vi "CSMsettings_ut_test.vi"(8 "Error In":errorcluster, 11 "CSMinfo in":T3={"Общие сведения"={"Регистрационный номер заказа"="", "Идентификация (шифр) образца"="", "IMEI образца"="", "НД, устанавливающий требования"="", "Методы испытаний (измерений)"="", "Дата начала испытаний"="", "Дата завершения испытаний"=""}, "Климатические условия внешней среды"={"Температура окружающего воздуха"="", "Относительная влажность воздуха"="", "Атмосферное давление"=""}, "Окно с настройками"={"Режим звонка связь"=0, "Напряжение источника"=0, "Условия окружающей среды"=0, "Номер образца"=0, "Источник питания"=0, "Номер испытания"=0, "Режим звонка тональный модем"=0, "Количество итераций TM"=100.0, "Аутентификация"=0, "Колличество повторов измерений"=1.0, "Сим карта"=0, "VISA adress of CMW500"="", "Input attenuation"=1.0, "Output attenuation"=1.0, "Call Release Type"=0, "GSM Band"=0, "BCCH Channel Number"=0.0, "TCH Channel Number"=0.0, "Codec"=0, "AWGN"=0, "snrRatioInDb"=0.0, "GSM Fading"=0, "UL C/I ratio"=0, "Use a custom network ID"=FALSE, "MCC (Mobile Country Code)"=0.0, "MNC (Mobile Network Code)"=0.0, "NCC (Network Color Code)"=0.0, "MNC digit count"=0, "BCC (Base station Color Code)"=0.0, "LAC (Location Area Code)"=0.0, "RAC (Routing Area Code)"=0.0, "Cell Identity"=0.0, "Override UE ID"=FALSE, "MCC (UE Mobile Country Code)"=0.0, "MNC (UE Mobile Network Code)"=0.0, "MSIN (Mobile Subscription ID)"=0.0, "InputScaleFactor"=0, "OutputScaleFactor"=0, "Post MSD wave file playback 3GPP  26.269 \nEU_DTMF_tones"=FALSE, "Scenario"=0, "AlAckBehavior"=0, "PSAP listens for PUSH"=FALSE, "BCCH Channel Power"=0.0, "TCH Channel Power"=0.0}} {"Окно с настройками"."AlAckBehavior" items=["POSITIVE", "CLEAR_DOWN", "LOOP_BACK_MSD_PART"]; "Окно с настройками"."Scenario" items=["NORMAL", "NORMAL_IMMEDIATE_START", "TIMEOUT_T3", "ALLRV_REQ", "SUPPRESS_MSD", "SUPPRESS_ALACK", "SUPPRESS_SEND_MSD"]; "Окно с настройками"."OutputScaleFactor" items=["ONE", "QUARTER", "HALF", "TWO", "FOUR"]; "Окно с настройками"."InputScaleFactor" items=["ONE", "QUARTER", "HALF", "TWO", "FOUR"]; "Окно с настройками"."MNC digit count" items=["TWO", "THREE"]; "Окно с настройками"."UL C/I ratio" items=["Ci1Db", "Ci4Db", "Ci7Db", "Ci10Db", "Ci13Db", "Ci16Db"]; "Окно с настройками"."GSM Fading" items=["GsmFadingOff", "GsmEtsiTs103412DlFading", "GsmEtsiTs103412UlFading", "GsmEtsiTs103412DlUlFading"]; "Окно с настройками"."AWGN" items=["Off", "50MhzAwgn"]; "Окно с настройками"."Codec" items=["FRV2", "AMRH_GMSK_7K95", "AMRH_GMSK_7K40", "AMRH_GMSK_6K70", "AMRH_GMSK_5K90", "AMRH_GMSK_5K15", "AMRH_GMSK_4K75", "AMRF_GMSK_12K20", "AMRF_GMSK_10K20", "AMRF_GMSK_7K95", "AMRF_GMSK_7K40 ", "AMRF_GMSK_6K70", "AMRF_GMSK_5K90", "AMRF_GMSK_5K15", "AMRF_GMSK_4K75", "FRV1", "HRV1", "WAMR_GMSK_6K60", "WAMR_GMSK_8K85", "WAMR_GMSK_12K65"]; "Окно с настройками"."GSM Band" items=["GSM450", "GSM850", "GSM900", "GSM1800", "GSM1900"]; "Окно с настройками"."Call Release Type" items=["NormalRelease", "CallInterruption"]; "Окно с настройками"."Сим карта" items=["SIM", "eSIM"]; "Окно с настройками"."Колличество повторов измерений" min=1.0 max=100.0 format="%#_3g"; "Окно с настройками"."Аутентификация" items=["On", "Off"]; "Окно с настройками"."Режим звонка тональный модем" items=["Автоматически (AT) GEMALTO", "Автоматически (AT) SIMCOM", "Автоматически (AT) TELIT", "Автоматически (AT) PROGRESS", "Автоматически (AT) PROGRESS GREEN", "Автоматически (AT) PROGRESS BLUE", "Автоматически (реле)", "Вручную"]; "Окно с настройками"."Номер испытания" items=["1", "2", "3"]; "Окно с настройками"."Источник питания" items=["Не используется", "IT6332A"]; "Окно с настройками"."Номер образца" items=["1", "2", "3"]; "Окно с настройками"."Условия окружающей среды" items=["UnormTnorm", "UminTmin", "UmaxTmin", "UminTmax", "UmaxTmax", "TypeA", "TypeB"]; "Окно с настройками"."Напряжение источника" items=["12", "24"]; "Окно с настройками"."Режим звонка связь" items=["Автоматически (AT) GEMALTO", "Автоматически (AT) SIMCOM", "Автоматически (AT) TELIT", "Автоматически (AT) PROGRESS", "Автоматически (AT) PROGRESS GREEN", "Автоматически (AT) PROGRESS BLUE", "Автоматически (реле)", "Вручную"]}) -> (0 "Error Out":errorcluster, 3 "CSMinfo out":T3={"Общие сведения"={"Регистрационный номер заказа"="", "Идентификация (шифр) образца"="", "IMEI образца"="", "НД, устанавливающий требования"="", "Методы испытаний (измерений)"="", "Дата начала испытаний"="", "Дата завершения испытаний"=""}, "Климатические условия внешней среды"={"Температура окружающего воздуха"="", "Относительная влажность воздуха"="", "Атмосферное давление"=""}, "Окно с настройками"={"Режим звонка связь"=0, "Напряжение источника"=0, "Условия окружающей среды"=0, "Номер образца"=0, "Источник питания"=0, "Номер испытания"=0, "Режим звонка тональный модем"=0, "Количество итераций TM"=0.0, "Аутентификация"=0, "Колличество повторов измерений"=1.0, "Сим карта"=0, "VISA adress of CMW500"="", "Input attenuation"=1.0, "Output attenuation"=1.0, "Call Release Type"=0, "GSM Band"=0, "BCCH Channel Number"=0.0, "TCH Channel Number"=0.0, "Codec"=0, "AWGN"=0, "snrRatioInDb"=0.0, "GSM Fading"=0, "UL C/I ratio"=0, "Use a custom network ID"=FALSE, "MCC (Mobile Country Code)"=0.0, "MNC (Mobile Network Code)"=0.0, "NCC (Network Color Code)"=0.0, "MNC digit count"=0, "BCC (Base station Color Code)"=0.0, "LAC (Location Area Code)"=0.0, "RAC (Routing Area Code)"=0.0, "Cell Identity"=0.0, "Override UE ID"=FALSE, "MCC (UE Mobile Country Code)"=0.0, "MNC (UE Mobile Network Code)"=0.0, "MSIN (Mobile Subscription ID)"=0.0, "InputScaleFactor"=0, "OutputScaleFactor"=0, "Post MSD wave file playback 3GPP  26.269 \nEU_DTMF_tones"=FALSE, "Scenario"=0, "AlAckBehavior"=0, "PSAP listens for PUSH"=FALSE, "BCCH Channel Power"=0.0, "TCH Channel Power"=0.0}} {"Окно с настройками"."AlAckBehavior" items=["POSITIVE", "CLEAR_DOWN", "LOOP_BACK_MSD_PART"]; "Окно с настройками"."Scenario" items=["NORMAL", "NORMAL_IMMEDIATE_START", "TIMEOUT_T3", "ALLRV_REQ", "SUPPRESS_MSD", "SUPPRESS_ALACK", "SUPPRESS_SEND_MSD"]; "Окно с настройками"."OutputScaleFactor" items=["ONE", "QUARTER", "HALF", "TWO", "FOUR"]; "Окно с настройками"."InputScaleFactor" items=["ONE", "QUARTER", "HALF", "TWO", "FOUR"]; "Окно с настройками"."MNC digit count" items=["TWO", "THREE"]; "Окно с настройками"."UL C/I ratio" items=["Ci1Db", "Ci4Db", "Ci7Db", "Ci10Db", "Ci13Db", "Ci16Db"]; "Окно с настройками"."GSM Fading" items=["GsmFadingOff", "GsmEtsiTs103412DlFading", "GsmEtsiTs103412UlFading", "GsmEtsiTs103412DlUlFading"]; "Окно с настройками"."AWGN" items=["Off", "50MhzAwgn"]; "Окно с настройками"."Codec" items=["FRV2", "AMRH_GMSK_7K95", "AMRH_GMSK_7K40", "AMRH_GMSK_6K70", "AMRH_GMSK_5K90", "AMRH_GMSK_5K15", "AMRH_GMSK_4K75", "AMRF_GMSK_12K20", "AMRF_GMSK_10K20", "AMRF_GMSK_7K95", "AMRF_GMSK_7K40 ", "AMRF_GMSK_6K70", "AMRF_GMSK_5K90", "AMRF_GMSK_5K15", "AMRF_GMSK_4K75", "FRV1", "HRV1", "WAMR_GMSK_6K60", "WAMR_GMSK_8K85", "WAMR_GMSK_12K65"]; "Окно с настройками"."GSM Band" items=["GSM450", "GSM850", "GSM900", "GSM1800", "GSM1900"]; "Окно с настройками"."Call Release Type" items=["NormalRelease", "CallInterruption"]; "Окно с настройками"."Сим карта" items=["SIM", "eSIM"]; "Окно с настройками"."Колличество повторов измерений" min=1.0 max=100.0 format="%#_3g"; "Окно с настройками"."Аутентификация" items=["On", "Off"]; "Окно с настройками"."Режим звонка тональный модем" items=["Автоматически (AT) GEMALTO", "Автоматически (AT) SIMCOM", "Автоматически (AT) TELIT", "Автоматически (AT) PROGRESS", "Автоматически (AT) PROGRESS GREEN", "Автоматически (AT) PROGRESS BLUE", "Автоматически (реле)", "Вручную"]; "Окно с настройками"."Номер испытания" items=["1", "2", "3"]; "Окно с настройками"."Источник питания" items=["Не используется", "IT6332A"]; "Окно с настройками"."Номер образца" items=["1", "2", "3"]; "Окно с настройками"."Условия окружающей среды" items=["UnormTnorm", "UminTmin", "UmaxTmin", "UminTmax", "UmaxTmax", "TypeA", "TypeB"]; "Окно с настройками"."Напряжение источника" items=["12", "24"]; "Окно с настройками"."Режим звонка связь" items=["Автоматически (AT) GEMALTO", "Автоматически (AT) SIMCOM", "Автоматически (AT) TELIT", "Автоматически (AT) PROGRESS", "Автоматически (AT) PROGRESS GREEN", "Автоматически (AT) PROGRESS BLUE", "Автоматически (реле)", "Вручную"]})   [LabVIEW 2018]
uses:
  CSMinfo.ctl
  MOKO_LabViewLibrary/MokoSTM/MokoClassicUtilitySTM/MCUS_STM.ctl
  MOKO_LabViewLibrary/MokoSTM/MokoClassicUtilitySTM/MCUS_ITEM.ctl
panel:
  in  "Применить":bool
  in  "Общие настройки/Настройки модема":T1(tab)
  in  "Сим карта":u16(ring) items=["SIM", "eSIM"]
  in  "Количество повторов измерений":dbl=1.0
  in  "Аунтетификация":u16(ring) items=["On", "Off"]
  in  "Количество итераций TM":dbl=100.0
  in  "Условия окружающей среды":u16(ring) items=["UnormTnorm", "UminTmin", "UmaxTmin", "UminTmax", "UmaxTmax", "TypeA", "TypeB"]
  in  "Режим звонка тональный модем":u16(ring) items=["Автоматически (AT) GEMALTO", "Автоматически (AT) SIMCOM", "Автоматически (AT) TELIT", "Автоматически (AT) PROGRESS", "Автоматически (AT) PROGRESS GREEN", "Автоматически (AT) PROGRESS BLUE", "Автоматически (реле)", "Вручную"]
  in  "Номер испытания":u16(ring) items=["1", "2", "3"]
  in  "Источник питания":u16(ring) items=["Не используется", "IT6332A"]
  in  "Напряжение источника":u16(ring) items=["12", "24"]
  in  "Номер образца":u16(ring) items=["1", "2", "3"]
  in  "Режим звонка связь":u16(ring) items=["Автоматически (AT) GEMALTO", "Автоматически (AT) SIMCOM", "Автоматически (AT) TELIT", "Автоматически (AT) PROGRESS", "Автоматически (AT) PROGRESS GREEN", "Автоматически (AT) PROGRESS BLUE", "Автоматически (реле)", "Вручную"]
  in  "Настройки модема по умолчанию":enum32{"CMW500", "GSM", "PSAP"}(tab)
  in  "VISA adress of CMW500":string="TCPIP0::169.254.98.10::inst0::INSTR"
  in  "Input attenuation":dbl=1.0
  in  "Output attenuation":dbl=100.0
  in  "GSM":T2(tab)
  in  "BCCH Channel Power":dbl=1.0
  in  "TCH Channel Power":dbl=1.0
  in  "GSM Band":u16(ring) items=["GSM450", "GSM850", "GSM900", "GSM1800", "GSM1900"]
  in  "BCCH Channel Number":dbl=1.0
  in  "TCH Channel number":dbl=1.0
  in  "Codec":u16(ring) items=["FRV2", "AMRH_GMSK_7K95", "AMRH_GMSK_7K40", "AMRH_GMSK_6K70", "AMRH_GMSK_5K90", "AMRH_GMSK_5K15", "AMRH_GMSK_4K75", "AMRF_GMSK_12K20", "AMRF_GMSK_10K20", "AMRF_GMSK_7K95", "AMRF_GMSK_7K40 ", "AMRF_GMSK_6K70", "AMRF_GMSK_5K90", "AMRF_GMSK_5K15", "AMRF_GMSK_4K75", "FRV1", "HRV1", "WAMR_GMSK_6K60", "WAMR_GMSK_8K85", "WAMR_GMSK_12K65"]
  in  "AWGN":u16(ring) items=["Off", "50MhzAwgn"]
  in  "snrRatioInDb":dbl=1.0
  in  "GSM Fading":u16(ring) items=["GsmFadingOff", "GsmEtsiTs103412DlFading", "GsmEtsiTs103412UlFading", "GsmEtsiTs103412DlUlFading"]
  in  "UL C/I ratio":u16(ring) items=["Ci1Db", "Ci4Db", "Ci7Db", "Ci10Db", "Ci13Db", "Ci16Db"]
  in  "MCC (Mobile Country Code)":dbl=1.0
  in  "Use a custom network ID":bool
  in  "MNC (Mobile Network Code)":dbl=1.0
  in  "MNC digit count":u16(ring) items=["TWO", "THREE"]
  in  "BCC (Base station Color Code)":dbl=1.0
  in  "NCC (Network Color Code)":dbl=1.0
  in  "RAC (Routing Area Code)":dbl=1.0
  in  "LAC (Location Area Code)":dbl=1.0
  in  "Cell Identity":dbl=1.0
  in  "Override UE ID":bool
  in  "MNC (UE Mobile Network Code)":dbl=1.0
  in  "MCC (UE Mobile Country Code)":dbl=1.0
  in  "MSIN (Mobile Subscription ID)":dbl=1.0 format="%#_10g"
  in  "Call Release Type":u16(ring) items=["NormalRelease", "CallInterruption"]
  in  "OutputScaleFactor":u16(ring) items=["ONE", "QUARTER", "HALF", "TWO", "FOUR"]
  in  "PSAP listens for PUSH":bool
  in  "AlAckBehavior":u16(ring) items=["POSITIVE", "CLEAR_DOWN", "LOOP_BACK_MSD_PART"]
  in  "Scenario":u16(ring) items=["NORMAL", "NORMAL_IMMEDIATE_START", "TIMEOUT_T3", "ALLRV_REQ", "SUPPRESS_MSD", "SUPPRESS_ALACK", "SUPPRESS_SEND_MSD"]
  in  "InputScaleFactor":u16(ring) items=["ONE", "QUARTER", "HALF", "TWO", "FOUR"]
  in  "Post MSD wave file playback 3GPP  26.269 EU_DTMF_tones":bool
  # "0,4\n0,6\n1\n1,5\n1,6\n2,5\n4"
  # "kPa\nbar\nkgf/cm2\nMPa"
  # "1. Общие настройки"
  # "Номер образца:"
  # "Номер испытания:"
  # "Режим измерения:"
  # "Источник питания:"
  # "Напряжение источника питания, B:"
  # "2. Настройки связи"
  # "Режим звонка:"
  # "Аунтетификация:"
  # "Сим карта:"
  # "Количество повторов измерений:"
  # "3. Настройки тонального модема"
  # "Режим звонка:"
  # "Количество итераций Tonal:"
  # "VISA adress of CMW500:"
  # "Input attenuation:"
  # "Output attenuation:"
  # "GSM Band:"
  # "BCCH Channel Power"
  # "TCH Channel Power"
  # "BCCH Channel Number"
  # "TCH Channel number"
  # "Codec"
  # "8.6.6"
  # "AWGN"
  # "snrRatioInDb"
  # "GSM Fading"
  # "UL C/I ratio"
  # "MCC (Mobile Country Code)"
  # "MNC (Mobile Network Code)"
  # "MNC digit count"
  # "NCC (Network Color Code)"
  # "BCC (Base station Color Code)"
  # "LAC (Location Area Code)"
  # "RAC (Routing Area Code)"
  # "Cell Identity"
  # "MCC (UE Mobile Country Code)"
  # "MNC (UE Mobile Network Code)"
  # "MSIN (Mobile Subscription ID)"
  # "Call Release Type:"
  # "8.6.6"
  # "InputScaleFactor"
  # "OutputScaleFactor"
  # "8.6.7"
  # "8.6.8 (Use parameter NORMAL_IMMEDIATE_START)"
  # "Scenario"
  # "8.6.9 (Use parameter LOOP_BACK_MSD_PART)"
  # "AlAckBehavior"
  # "1. Общие настройки"
  # "Настройки модема по умолчанию"
  # "CMW500"
  # "PSAP"
  # "8.6.6"
  # "8.6.7"
  # "GSM"
  # "2. Настройки связи"
  # "8.6.8 (Use parameter NORMAL_IMMEDIATE_START)"
  # "8.6.9 (Use parameter LOOP_BACK_MSD_PART)"
  # "8.6.6"
  # "3. Настройки тонального модема"
  # "1. Общие настройки"
  # "Настройки модема по умолчанию"
  # "CMW500"
  # "PSAP"
  # "8.6.6"
  # "8.6.7"
  # "GSM"
  # "2. Настройки связи"
  # "8.6.8 (Use parameter NORMAL_IMMEDIATE_START)"
  # "8.6.9 (Use parameter LOOP_BACK_MSD_PART)"
  # "8.6.6"
  # "3. Настройки тонального модема"
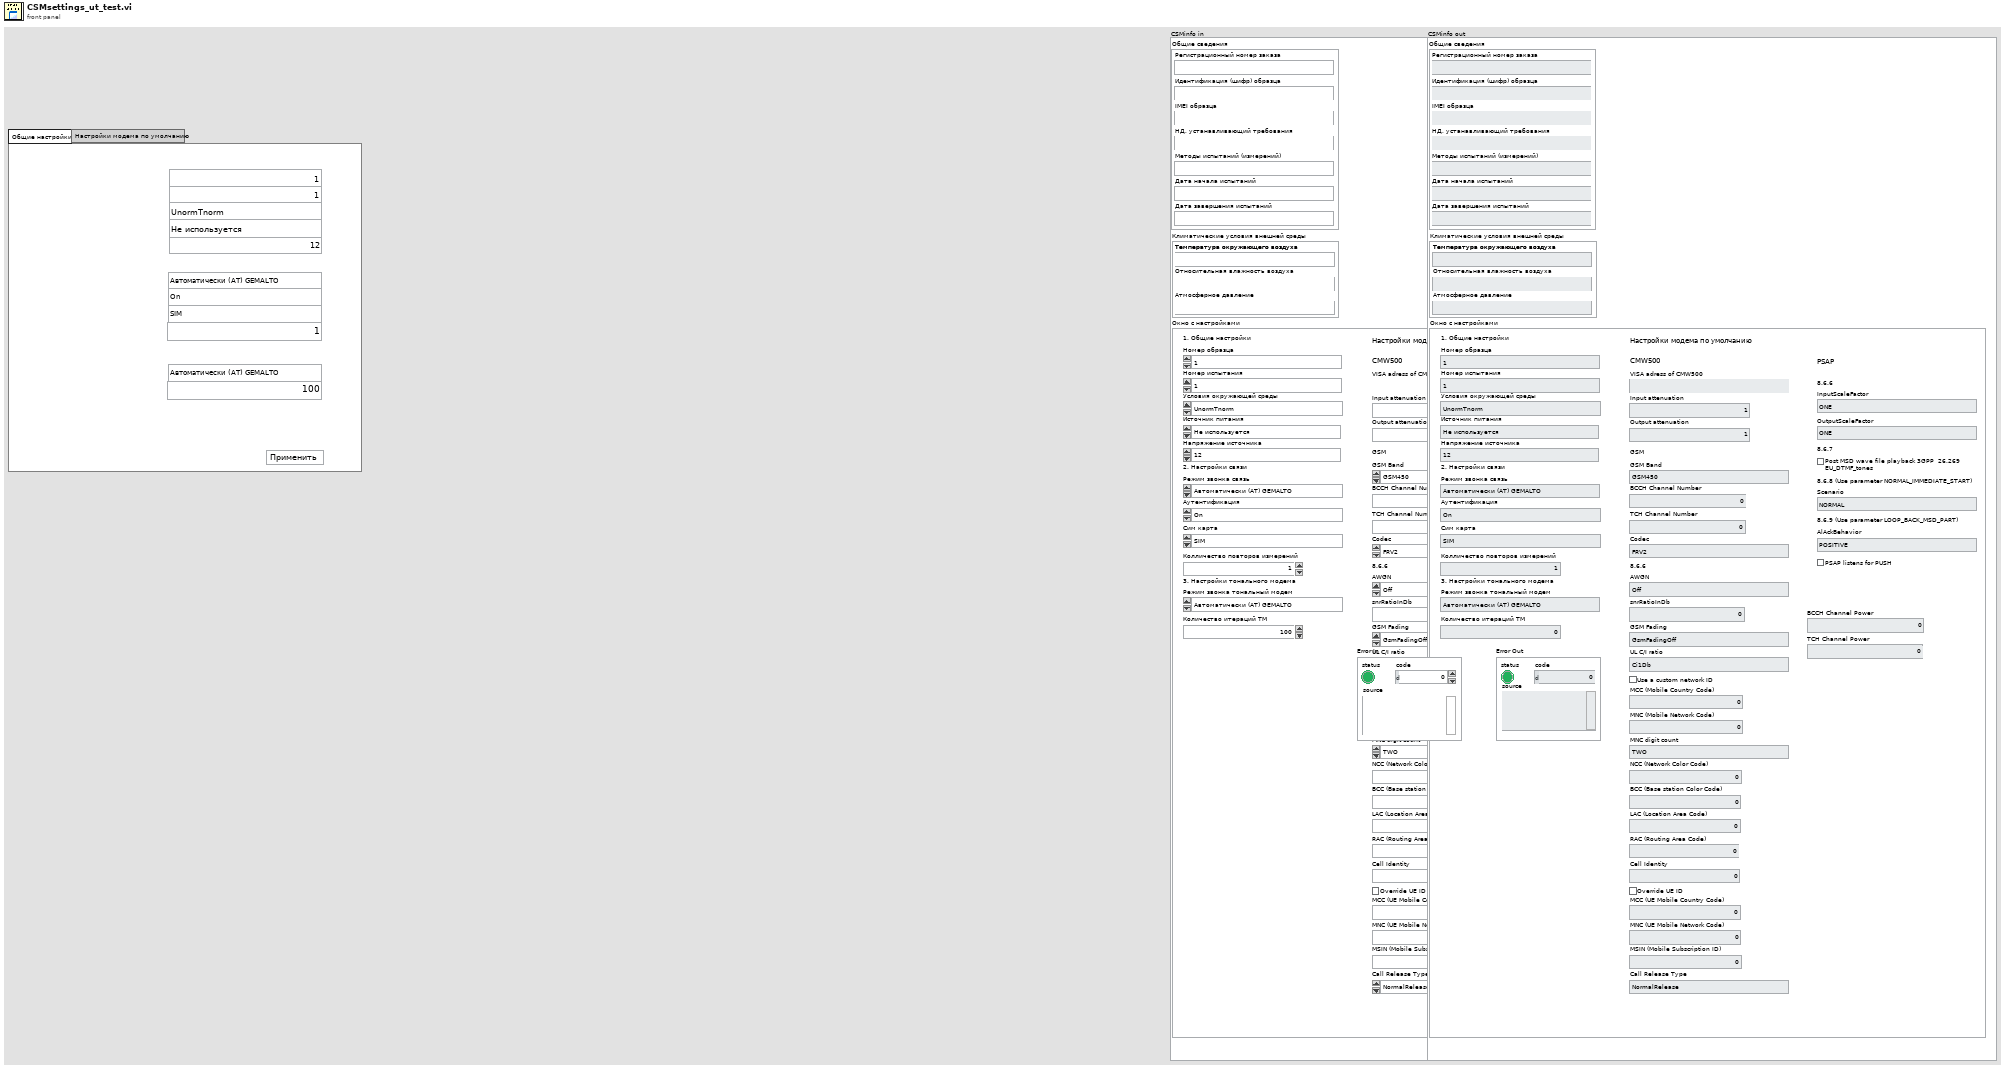
[diagram p1: front panel]
types:
  T1 = enum32{"Общие настройки", "Настройки модема по умолчанию"}
  T2 = enum32{"GSM Band/AWGN", "Custom network ID", "Call Release Type"}
  T3 = typedef "CSMinfo.ctl" = cluster{"Общие сведения":cluster{"Регистрационный номер заказа":string, "Идентификация (шифр) образца":string, "IMEI образца":string, "НД, устанавливающий требования":string, "Методы испытаний (измерений)":string, "Дата начала испытаний":string, "Дата завершения испытаний":string}, "Климатические условия внешней среды":cluster{"Температура окружающего воздуха":string, "Относительная влажность воздуха":string, "Атмосферное давление":string}, "Окно с настройками":cluster{"Режим звонка связь":u16, "Напряжение источника":u16, "Условия окружающей среды":u16, "Номер образца":u16, "Источник питания":u16, "Номер испытания":u16, "Режим звонка тональный модем":u16, "Количество итераций TM":dbl, "Аутентификация":u16, "Колличество повторов измерений":dbl, "Сим карта":u16, "VISA adress of CMW500":string, "Input attenuation":dbl, "Output attenuation":dbl, "Call Release Type":u16, "GSM Band":u16, "BCCH Channel Number":dbl, "TCH Channel Number":dbl, "Codec":u16, "AWGN":u16, "snrRatioInDb":dbl, "GSM Fading":u16, "UL C/I ratio":u16, "Use a custom network ID":bool, "MCC (Mobile Country Code)":dbl, "MNC (Mobile Network Code)":dbl, "NCC (Network Color Code)":dbl, "MNC digit count":u16, "BCC (Base station Color Code)":dbl, "LAC (Location Area Code)":dbl, "RAC (Routing Area Code)":dbl, "Cell Identity":dbl, "Override UE ID":bool, "MCC (UE Mobile Country Code)":dbl, "MNC (UE Mobile Network Code)":dbl, "MSIN (Mobile Subscription ID)":dbl, "InputScaleFactor":u16, "OutputScaleFactor":u16, "Post MSD wave file playback 3GPP  26.269 \nEU_DTMF_tones":bool, "Scenario":u16, "AlAckBehavior":u16, "PSAP listens for PUSH":bool, "BCCH Channel Power":dbl, "TCH Channel Power":dbl}}
  T4 = typedef "MCUS_STM.ctl" = cluster{"main stm":T5, "data":string}
  T5 = typedef "MCUS_ITEM.ctl" = enum16{"idle", "_____ main_____ ", "Init", "Stop", "Apply values"}
  T6 = typedef "LVStringsAndValuesArrayTypeDef_U16.ctl" = cluster{"String":string, "Value":u16}[]
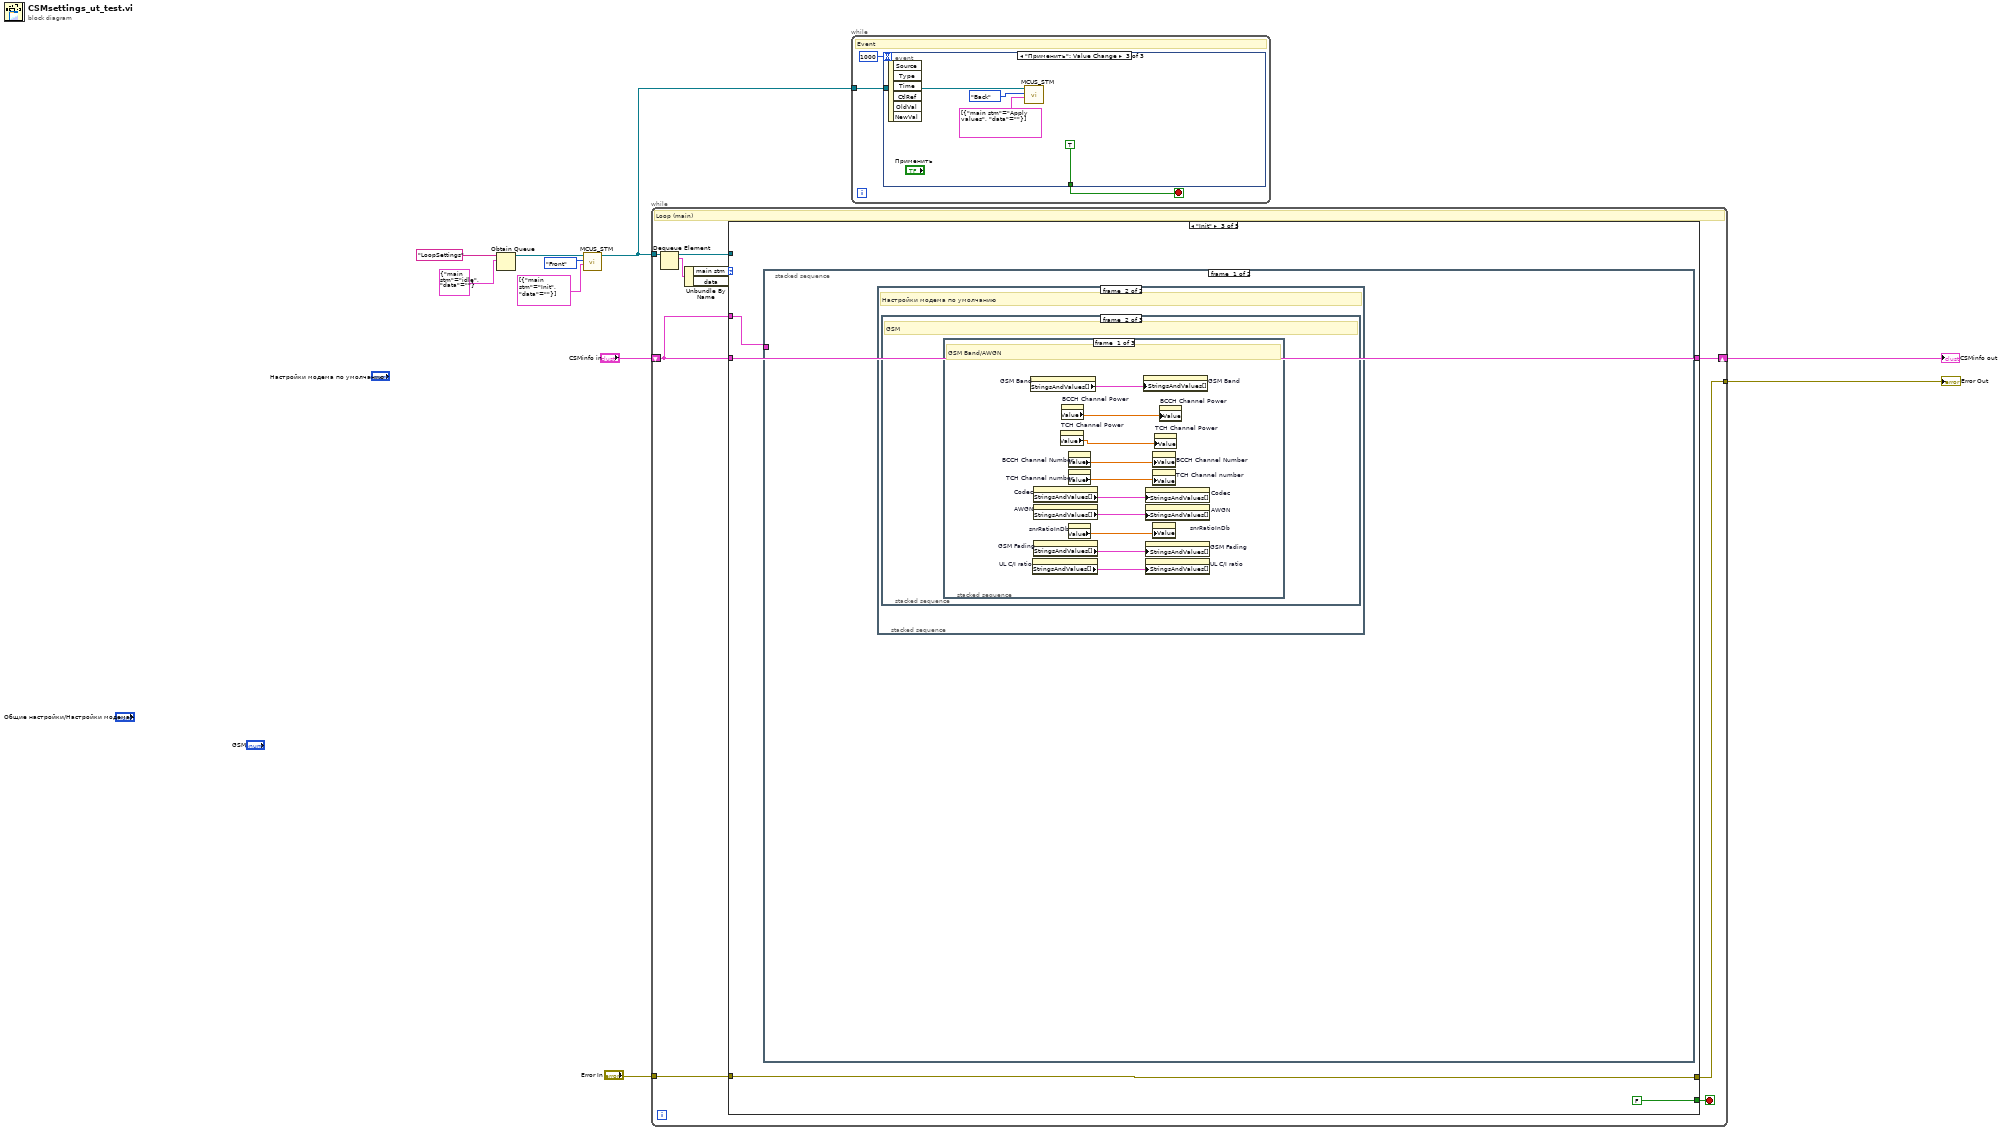
[diagram p0: block diagram]
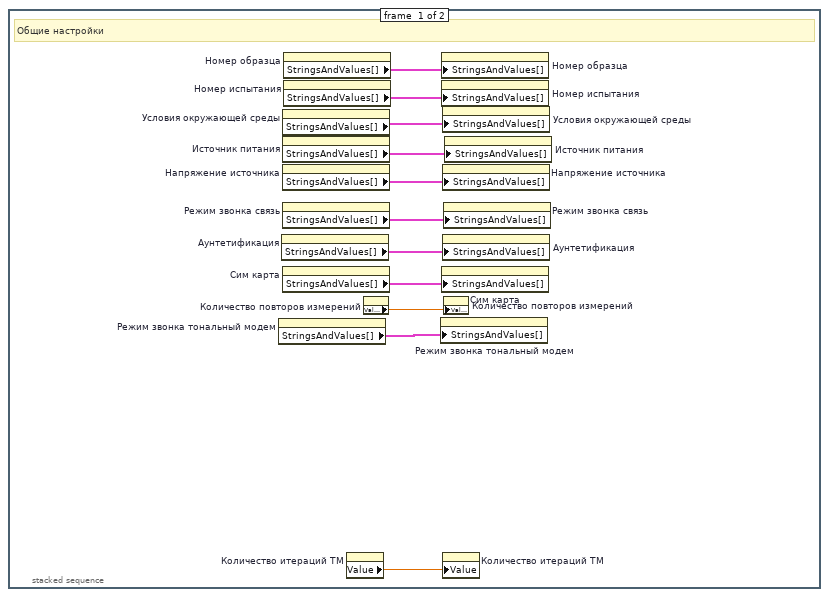
[diagram p4: hidden frame]
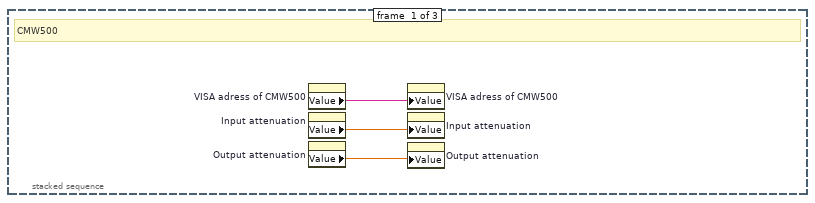
[diagram p5: hidden frame]
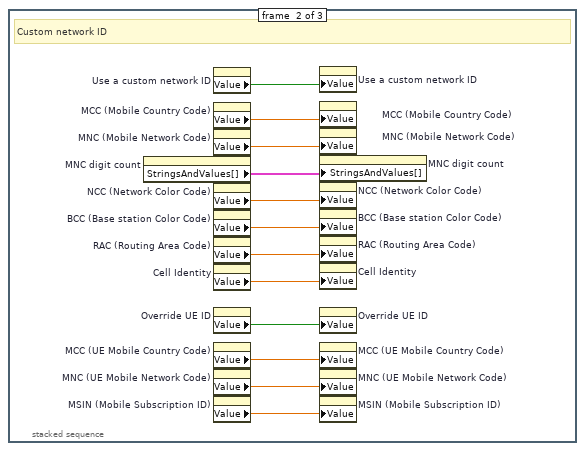
[diagram p6: hidden frame]
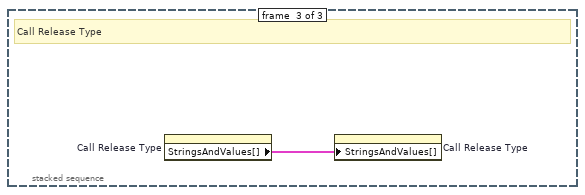
[diagram p7: hidden frame]
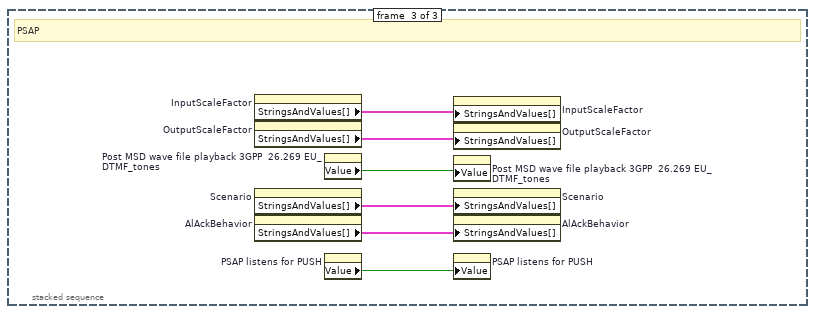
[diagram p8: hidden frame]
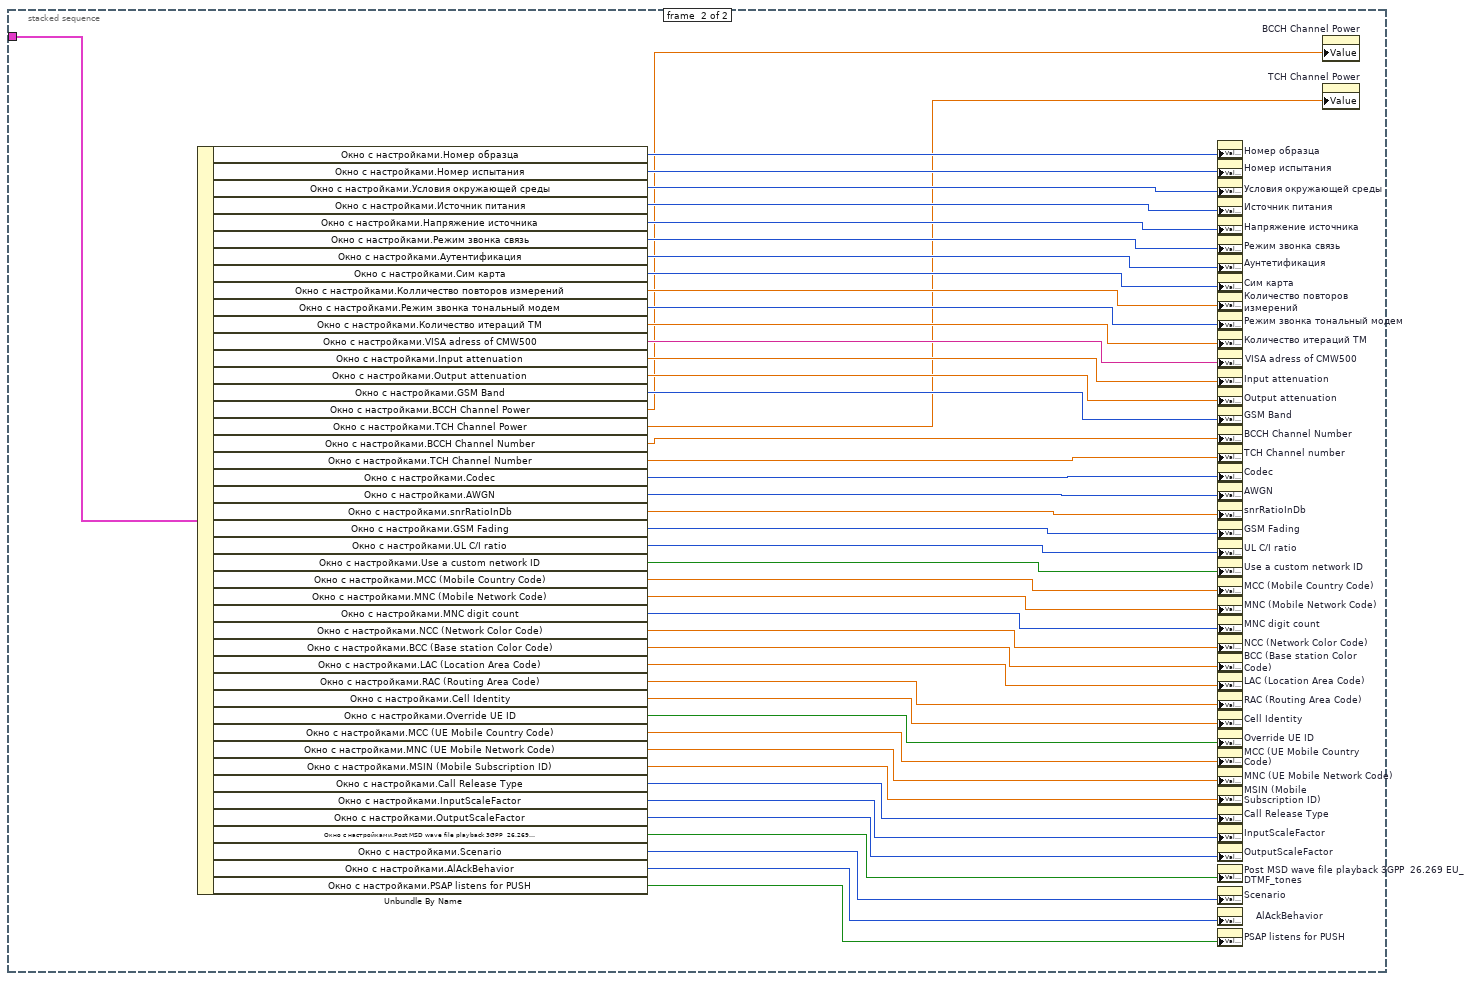
[diagram p9: hidden frame]
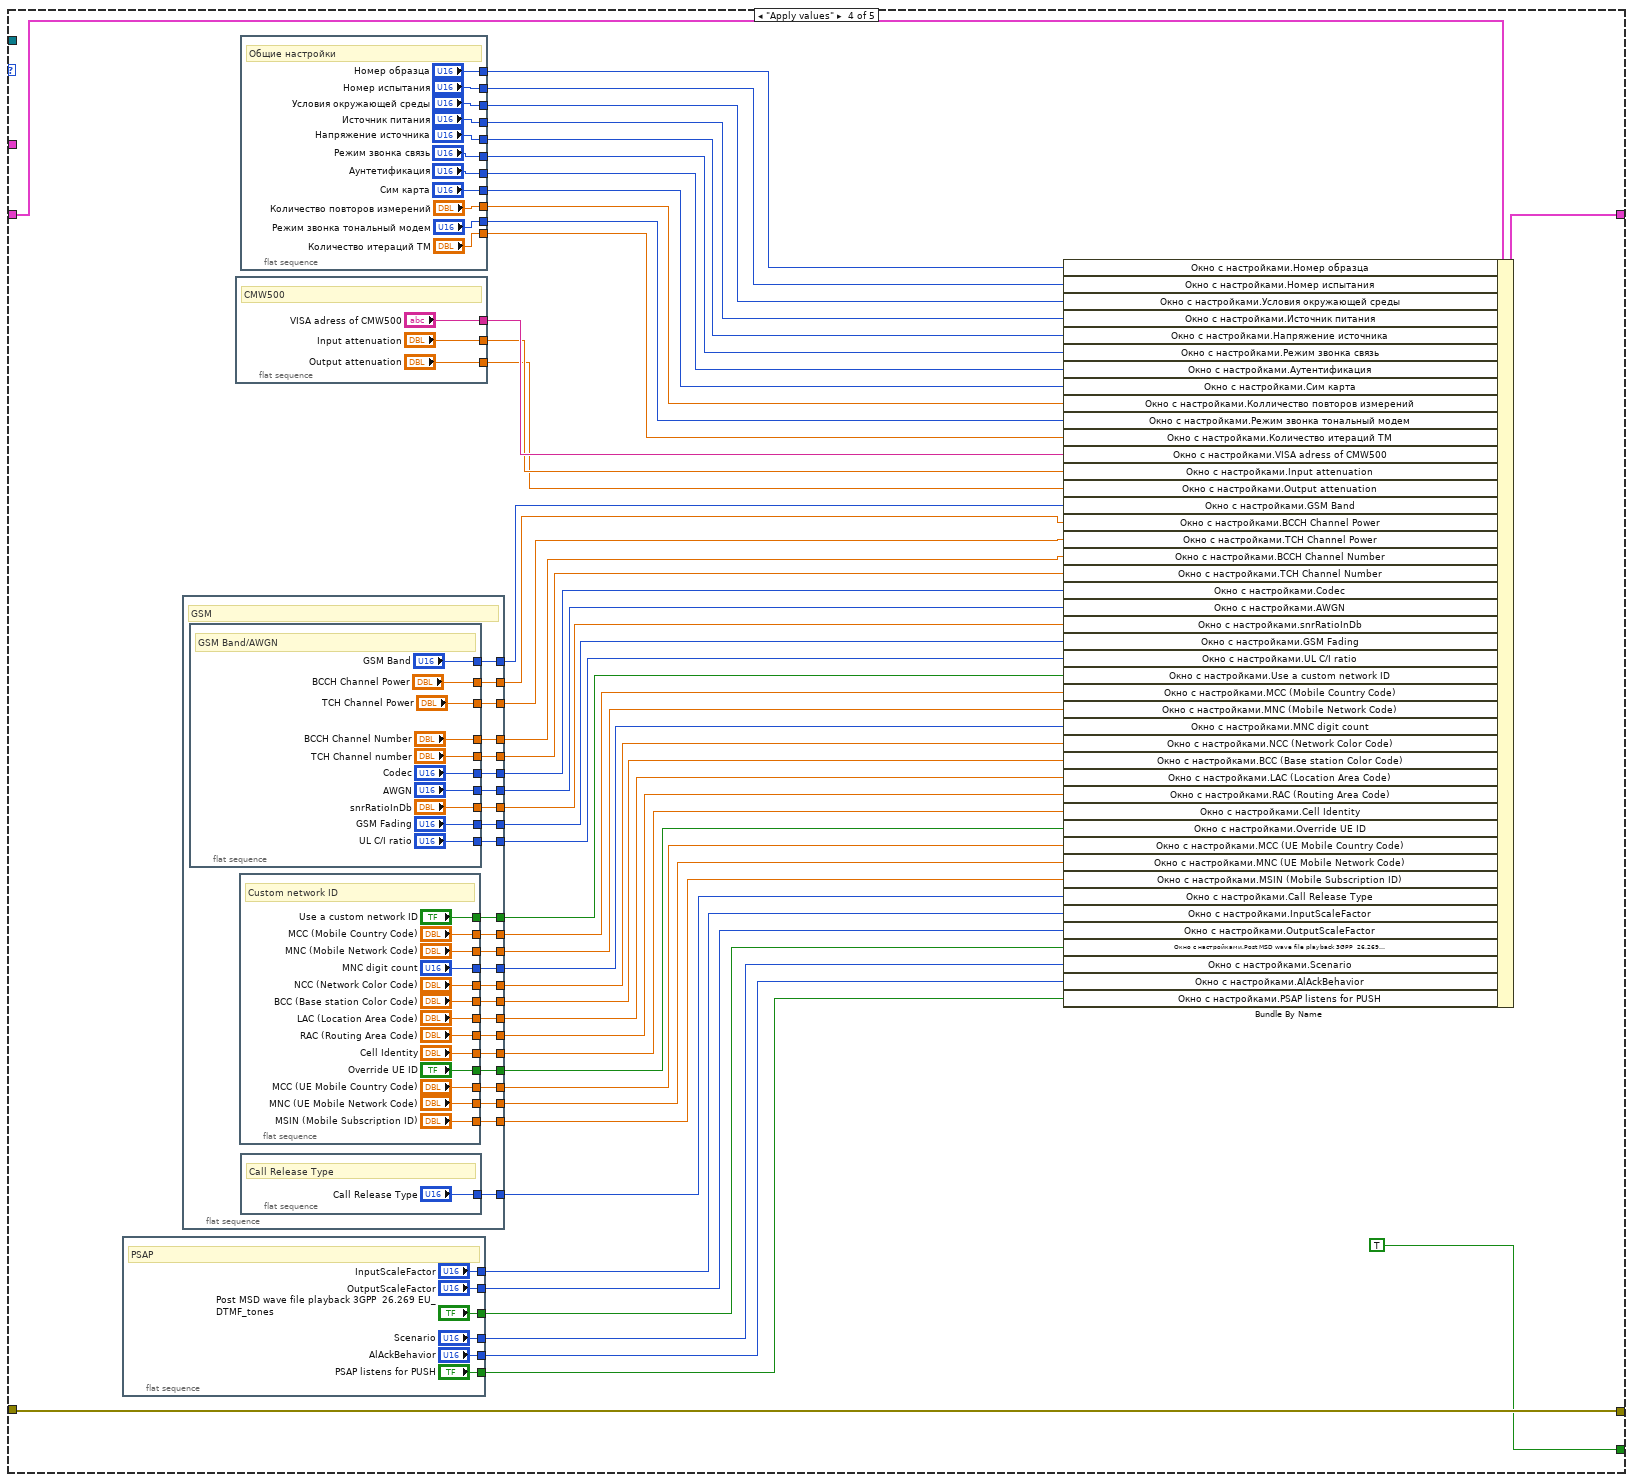
[diagram p10: hidden frame]
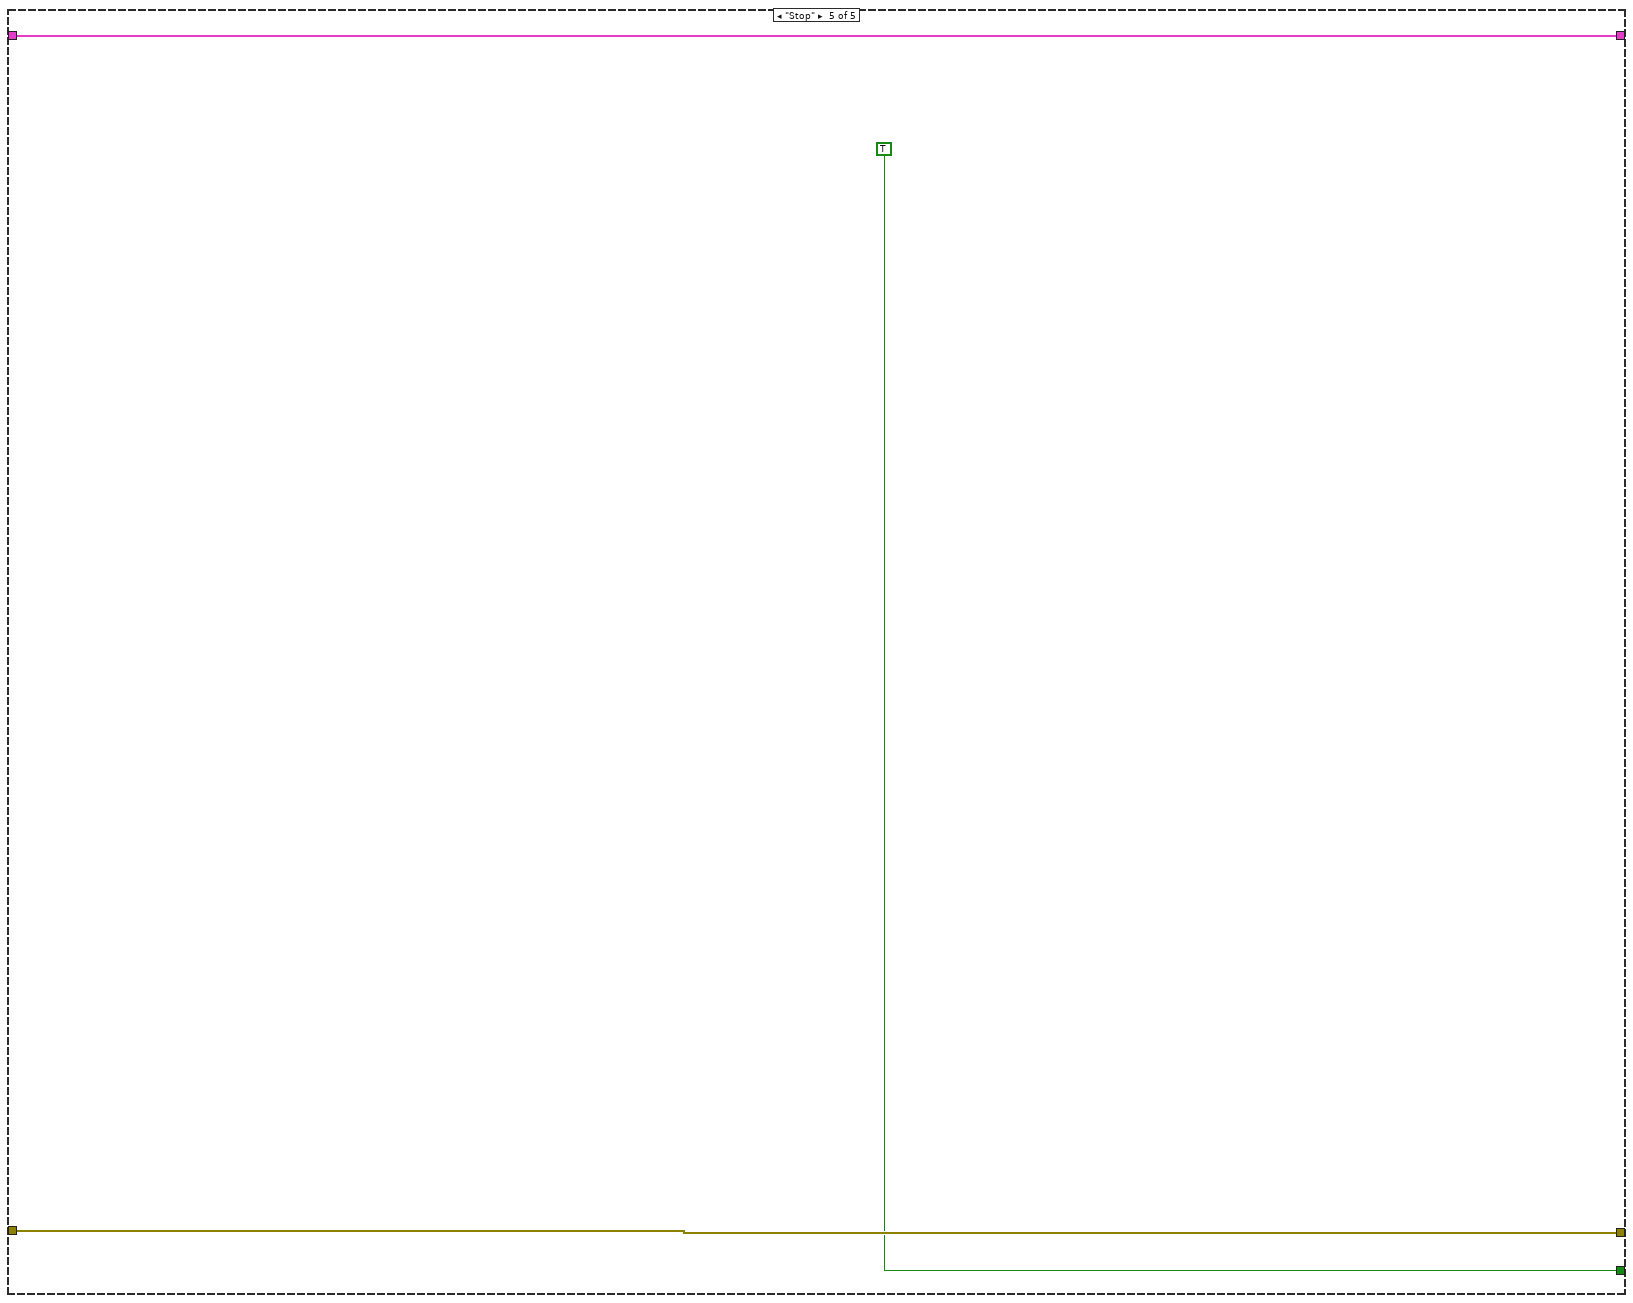
[diagram p11: hidden frame]
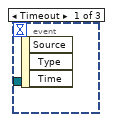
[diagram p12: hidden frame]
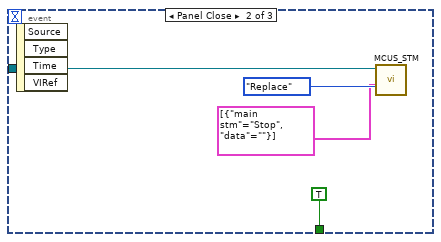
[diagram p13: hidden frame]
diagram:
  n1 = Obtain Queue(name (unnamed)="LoopSettings", element data type=T4 {"main stm"=enum."idle", "data"=""} ("MOKO_NMEA")) -> (queue out=w10:refnum<queue>)  [unwired: 3 in, 2 out]
  n2 = call "MCUS_STM.vi"("StateMachineSteps"=T4[] [{"main stm"=enum."Init", "data"=""}], "FNs"=enum16{"Back", "Front", "Replace"}."Front", "Queue in"=w10) -> ("Queue out"=w5:refnum<queue>)  [unwired: 7 in, 1 out]
  n3 = while {
    tunnel: w5 -> [w19]
    tunnel: "Error In" -> [w14]
    tunnel: [w13] -> w3
    shift-right: [w12] -> w1
    shift-left: "CSMinfo in" -> [w11]
    stop <- w15 stop-if-true
    # "Loop (main)"
    n4 = Dequeue Element(queue=w19) -> (queue out=w18:refnum<queue>, element=w17:T4)  [unwired: 2 in, 2 out]
    n5 = Unbundle By Name(w17) -> ("main stm"=w16:T5)  [unwired: 1 out]
    n6 = case shown="\"Init\"" w16 {
      tunnel: w18 -> [_ _ _ _ _]
      tunnel: [_ _ FALSE TRUE TRUE] -> w15
      tunnel: w14 -> [w20 w22 w27 w163 w234]
      tunnel: [w20 w22 w27 w163 w234] -> w13
      tunnel: [w21 w23 w25 w160 w233] -> w12
      tunnel: w11 -> [w21 w23 w25 w161 w233]
      tunnel: w11 -> [_ _ w24 _ _]
      frame "idle", Default {
      }
      frame "_____ main_____ " {
      }
      frame "Init" {
        n7 = stacked-sequence {
          tunnel: w24 -> [_ w115]
          frame #0 {
            n8 = stacked-sequence {
              frame #0 {
                # "Общие настройки"
                n9 = property on="Режим звонка тональный модем" class="Ring (strict)"() -> ("StringsAndValues[]"=w29:T6)  [unwired: 2 in, 2 out]
                n10 = property on="Аунтетификация" class="Ring (strict)"() -> ("StringsAndValues[]"=w36:T6)  [unwired: 2 in, 2 out]
                n11 = property on="Условия окружающей среды" class="Ring (strict)"() -> ("StringsAndValues[]"=w34:T6)  [unwired: 2 in, 2 out]
                n12 = property on="Источник питания" class="Ring (strict)"() -> ("StringsAndValues[]"=w35:T6)  [unwired: 2 in, 2 out]
                n13 = property on="Напряжение источника" class="Ring (strict)"() -> ("StringsAndValues[]"=w33:T6)  [unwired: 2 in, 2 out]
                n14 = property on="Режим звонка связь" class="Ring (strict)"() -> ("StringsAndValues[]"=w30:T6)  [unwired: 2 in, 2 out]
                n15 = property on="Сим карта" class="Ring (strict)"() -> ("StringsAndValues[]"=w38:T6)  [unwired: 2 in, 2 out]
                n16 = property on="Номер образца" class="Ring (strict)"() -> ("StringsAndValues[]"=w32:T6)  [unwired: 2 in, 2 out]
                n17 = property on="Номер испытания" class="Ring (strict)"() -> ("StringsAndValues[]"=w31:T6)  [unwired: 2 in, 2 out]
                n18 = property on="Количество итераций TM" class="DigNum (strict)"() -> ("Value"=w28:dbl)  [unwired: 2 in, 2 out]
                n19 = property on="Количество повторов измерений" class="DigNum (strict)"() -> ("Value"=w37:dbl)  [unwired: 2 in, 2 out]
                n20 = property on="Режим звонка тональный модем" class="Ring (strict)"("StringsAndValues[]"=w29) -> ()  [unwired: 2 in, 2 out]
                n21 = property on="Номер образца" class="Ring (strict)"("StringsAndValues[]"=w32) -> ()  [unwired: 2 in, 2 out]
                n22 = property on="Номер испытания" class="Ring (strict)"("StringsAndValues[]"=w31) -> ()  [unwired: 2 in, 2 out]
                n23 = property on="Сим карта" class="Ring (strict)"("StringsAndValues[]"=w38) -> ()  [unwired: 2 in, 2 out]
                n24 = property on="Условия окружающей среды" class="Ring (strict)"("StringsAndValues[]"=w34) -> ()  [unwired: 2 in, 2 out]
                n25 = property on="Напряжение источника" class="Ring (strict)"("StringsAndValues[]"=w33) -> ()  [unwired: 2 in, 2 out]
                n26 = property on="Аунтетификация" class="Ring (strict)"("StringsAndValues[]"=w36) -> ()  [unwired: 2 in, 2 out]
                n27 = property on="Количество итераций TM" class="DigNum (strict)"("Value"=w28) -> ()  [unwired: 2 in, 2 out]
                n28 = property on="Режим звонка связь" class="Ring (strict)"("StringsAndValues[]"=w30) -> ()  [unwired: 2 in, 2 out]
                n29 = property on="Количество повторов измерений" class="DigNum (strict)"("Value"=w37) -> ()  [unwired: 2 in, 2 out]
                n30 = property on="Источник питания" class="Ring (strict)"("StringsAndValues[]"=w35) -> ()  [unwired: 2 in, 2 out]
              }
              frame #1 {
                # "Настройки модема по умолчанию"
                n31 = stacked-sequence {
                  frame #0 {
                    # "CMW500"
                    n32 = property on="VISA adress of CMW500" class="Str"() -> ("Value"=w39:string)  [unwired: 2 in, 2 out]
                    n33 = property on="Input attenuation" class="DigNum (strict)"() -> ("Value"=w40:dbl)  [unwired: 2 in, 2 out]
                    n34 = property on="Output attenuation" class="DigNum (strict)"() -> ("Value"=w41:dbl)  [unwired: 2 in, 2 out]
                    n35 = property on="VISA adress of CMW500" class="Str"("Value"=w39) -> ()  [unwired: 2 in, 2 out]
                    n36 = property on="Input attenuation" class="DigNum (strict)"("Value"=w40) -> ()  [unwired: 2 in, 2 out]
                    n37 = property on="Output attenuation" class="DigNum (strict)"("Value"=w41) -> ()  [unwired: 2 in, 2 out]
                  }
                  frame #1 {
                    # "GSM"
                    n38 = stacked-sequence {
                      frame #0 {
                        # "GSM Band/AWGN"
                        n39 = property on="GSM Band" class="Ring (strict)"() -> ("StringsAndValues[]"=w51:T6)  [unwired: 2 in, 2 out]
                        n40 = property on="UL C/I ratio" class="Ring (strict)"() -> ("StringsAndValues[]"=w44:T6)  [unwired: 2 in, 2 out]
                        n41 = property on="Codec" class="Ring (strict)"() -> ("StringsAndValues[]"=w48:T6)  [unwired: 2 in, 2 out]
                        n42 = property on="AWGN" class="Ring (strict)"() -> ("StringsAndValues[]"=w47:T6)  [unwired: 2 in, 2 out]
                        n43 = property on="GSM Fading" class="Ring (strict)"() -> ("StringsAndValues[]"=w45:T6)  [unwired: 2 in, 2 out]
                        n44 = property on="TCH Channel Power" class="DigNum (strict)"() -> ("Value"=w42:dbl)  [unwired: 2 in, 2 out]
                        n45 = property on="BCCH Channel Power" class="DigNum (strict)"() -> ("Value"=w43:dbl)  [unwired: 2 in, 2 out]
                        n46 = property on="BCCH Channel Number" class="DigNum (strict)"() -> ("Value"=w50:dbl)  [unwired: 2 in, 2 out]
                        n47 = property on="TCH Channel number" class="DigNum (strict)"() -> ("Value"=w49:dbl)  [unwired: 2 in, 2 out]
                        n48 = property on="snrRatioInDb" class="DigNum (strict)"() -> ("Value"=w46:dbl)  [unwired: 2 in, 2 out]
                        n49 = property on="GSM Band" class="Ring (strict)"("StringsAndValues[]"=w51) -> ()  [unwired: 2 in, 2 out]
                        n50 = property on="GSM Fading" class="Ring (strict)"("StringsAndValues[]"=w45) -> ()  [unwired: 2 in, 2 out]
                        n51 = property on="UL C/I ratio" class="Ring (strict)"("StringsAndValues[]"=w44) -> ()  [unwired: 2 in, 2 out]
                        n52 = property on="Codec" class="Ring (strict)"("StringsAndValues[]"=w48) -> ()  [unwired: 2 in, 2 out]
                        n53 = property on="AWGN" class="Ring (strict)"("StringsAndValues[]"=w47) -> ()  [unwired: 2 in, 2 out]
                        n54 = property on="BCCH Channel Number" class="DigNum (strict)"("Value"=w50) -> ()  [unwired: 2 in, 2 out]
                        n55 = property on="TCH Channel number" class="DigNum (strict)"("Value"=w49) -> ()  [unwired: 2 in, 2 out]
                        n56 = property on="snrRatioInDb" class="DigNum (strict)"("Value"=w46) -> ()  [unwired: 2 in, 2 out]
                        n57 = property on="TCH Channel Power" class="DigNum (strict)"("Value"=w42) -> ()  [unwired: 2 in, 2 out]
                        n58 = property on="BCCH Channel Power" class="DigNum (strict)"("Value"=w43) -> ()  [unwired: 2 in, 2 out]
                      }
                      frame #1 {
                        # "Custom network ID"
                        n59 = property on="MNC digit count" class="Ring (strict)"() -> ("StringsAndValues[]"=w60:T6)  [unwired: 2 in, 2 out]
                        n60 = property on="Use a custom network ID" class="Bool (strict)"() -> ("Value"=w63:bool)  [unwired: 2 in, 2 out]
                        n61 = property on="MCC (Mobile Country Code)" class="DigNum (strict)"() -> ("Value"=w62:dbl)  [unwired: 2 in, 2 out]
                        n62 = property on="MNC (Mobile Network Code)" class="DigNum (strict)"() -> ("Value"=w61:dbl)  [unwired: 2 in, 2 out]
                        n63 = property on="NCC (Network Color Code)" class="DigNum (strict)"() -> ("Value"=w59:dbl)  [unwired: 2 in, 2 out]
                        n64 = property on="BCC (Base station Color Code)" class="DigNum (strict)"() -> ("Value"=w58:dbl)  [unwired: 2 in, 2 out]
                        n65 = property on="RAC (Routing Area Code)" class="DigNum (strict)"() -> ("Value"=w57:dbl)  [unwired: 2 in, 2 out]
                        n66 = property on="Cell Identity" class="DigNum (strict)"() -> ("Value"=w56:dbl)  [unwired: 2 in, 2 out]
                        n67 = property on="Override UE ID" class="Bool (strict)"() -> ("Value"=w55:bool)  [unwired: 2 in, 2 out]
                        n68 = property on="MCC (UE Mobile Country Code)" class="DigNum (strict)"() -> ("Value"=w54:dbl)  [unwired: 2 in, 2 out]
                        n69 = property on="MNC (UE Mobile Network Code)" class="DigNum (strict)"() -> ("Value"=w53:dbl)  [unwired: 2 in, 2 out]
                        n70 = property on="MSIN (Mobile Subscription ID)" class="DigNum (strict)"() -> ("Value"=w52:dbl)  [unwired: 2 in, 2 out]
                        n71 = property on="Use a custom network ID" class="Bool (strict)"("Value"=w63) -> ()  [unwired: 2 in, 2 out]
                        n72 = property on="MCC (Mobile Country Code)" class="DigNum (strict)"("Value"=w62) -> ()  [unwired: 2 in, 2 out]
                        n73 = property on="MNC (Mobile Network Code)" class="DigNum (strict)"("Value"=w61) -> ()  [unwired: 2 in, 2 out]
                        n74 = property on="MNC digit count" class="Ring (strict)"("StringsAndValues[]"=w60) -> ()  [unwired: 2 in, 2 out]
                        n75 = property on="NCC (Network Color Code)" class="DigNum (strict)"("Value"=w59) -> ()  [unwired: 2 in, 2 out]
                        n76 = property on="BCC (Base station Color Code)" class="DigNum (strict)"("Value"=w58) -> ()  [unwired: 2 in, 2 out]
                        n77 = property on="RAC (Routing Area Code)" class="DigNum (strict)"("Value"=w57) -> ()  [unwired: 2 in, 2 out]
                        n78 = property on="Cell Identity" class="DigNum (strict)"("Value"=w56) -> ()  [unwired: 2 in, 2 out]
                        n79 = property on="Override UE ID" class="Bool (strict)"("Value"=w55) -> ()  [unwired: 2 in, 2 out]
                        n80 = property on="MCC (UE Mobile Country Code)" class="DigNum (strict)"("Value"=w54) -> ()  [unwired: 2 in, 2 out]
                        n81 = property on="MNC (UE Mobile Network Code)" class="DigNum (strict)"("Value"=w53) -> ()  [unwired: 2 in, 2 out]
                        n82 = property on="MSIN (Mobile Subscription ID)" class="DigNum (strict)"("Value"=w52) -> ()  [unwired: 2 in, 2 out]
                      }
                      frame #2 {
                        # "Call Release Type"
                        n83 = property on="Call Release Type" class="Ring (strict)"() -> ("StringsAndValues[]"=w64:T6)  [unwired: 2 in, 2 out]
                        n84 = property on="Call Release Type" class="Ring (strict)"("StringsAndValues[]"=w64) -> ()  [unwired: 2 in, 2 out]
                      }
                    }
                  }
                  frame #2 {
                    # "PSAP"
                    n85 = property on="InputScaleFactor" class="Ring (strict)"() -> ("StringsAndValues[]"=w70:T6)  [unwired: 2 in, 2 out]
                    n86 = property on="OutputScaleFactor" class="Ring (strict)"() -> ("StringsAndValues[]"=w69:T6)  [unwired: 2 in, 2 out]
                    n87 = property on="Scenario" class="Ring (strict)"() -> ("StringsAndValues[]"=w67:T6)  [unwired: 2 in, 2 out]
                    n88 = property on="AlAckBehavior" class="Ring (strict)"() -> ("StringsAndValues[]"=w66:T6)  [unwired: 2 in, 2 out]
                    n89 = property on="Post MSD wave file playback 3GPP  26.269 EU_DTMF_tones" class="Bool (strict)"() -> ("Value"=w68:bool)  [unwired: 2 in, 2 out]
                    n90 = property on="PSAP listens for PUSH" class="Bool (strict)"() -> ("Value"=w65:bool)  [unwired: 2 in, 2 out]
                    n91 = property on="InputScaleFactor" class="Ring (strict)"("StringsAndValues[]"=w70) -> ()  [unwired: 2 in, 2 out]
                    n92 = property on="OutputScaleFactor" class="Ring (strict)"("StringsAndValues[]"=w69) -> ()  [unwired: 2 in, 2 out]
                    n93 = property on="Post MSD wave file playback 3GPP  26.269 EU_DTMF_tones" class="Bool (strict)"("Value"=w68) -> ()  [unwired: 2 in, 2 out]
                    n94 = property on="Scenario" class="Ring (strict)"("StringsAndValues[]"=w67) -> ()  [unwired: 2 in, 2 out]
                    n95 = property on="AlAckBehavior" class="Ring (strict)"("StringsAndValues[]"=w66) -> ()  [unwired: 2 in, 2 out]
                    n96 = property on="PSAP listens for PUSH" class="Bool (strict)"("Value"=w65) -> ()  [unwired: 2 in, 2 out]
                  }
                }
              }
            }
          }
          frame #1 {
            n97 = Unbundle By Name(w115) -> ("Окно с настройками.Номер образца"=w114:u16, "Окно с настройками.Номер испытания"=w113:u16, "Окно с настройками.Условия окружающей среды"=w112:u16, "Окно с настройками.Источник питания"=w111:u16, "Окно с настройками.Напряжение источника"=w110:u16, "Окно с настройками.Режим звонка связь"=w109:u16, "Окно с настройками.Аутентификация"=w106:u16, "Окно с настройками.Сим карта"=w104:u16, "Окно с настройками.Колличество повторов измерений"=w105:dbl, "Окно с настройками.Режим звонка тональный модем"=w108:u16, "Окно с настройками.Количество итераций TM"=w107:dbl, "Окно с настройками.VISA adress of CMW500"=w103:string, "Окно с настройками.Input attenuation"=w102:dbl, "Окно с настройками.Output attenuation"=w101:dbl, "Окно с настройками.GSM Band"=w100:u16, "Окно с настройками.BCCH Channel Power"=w72:dbl, "Окно с настройками.TCH Channel Power"=w71:dbl, "Окно с настройками.BCCH Channel Number"=w73:dbl, "Окно с настройками.TCH Channel Number"=w99:dbl, "Окно с настройками.Codec"=w98:u16, "Окно с настройками.AWGN"=w97:u16, "Окно с настройками.snrRatioInDb"=w96:dbl, "Окно с настройками.GSM Fading"=w95:u16, "Окно с настройками.UL C/I ratio"=w94:u16, "Окно с настройками.Use a custom network ID"=w93:bool, "Окно с настройками.MCC (Mobile Country Code)"=w92:dbl, "Окно с настройками.MNC (Mobile Network Code)"=w91:dbl, "Окно с настройками.MNC digit count"=w90:u16, "Окно с настройками.NCC (Network Color Code)"=w89:dbl, "Окно с настройками.BCC (Base station Color Code)"=w88:dbl, "Окно с настройками.LAC (Location Area Code)"=w87:dbl, "Окно с настройками.RAC (Routing Area Code)"=w86:dbl, "Окно с настройками.Cell Identity"=w85:dbl, "Окно с настройками.Override UE ID"=w84:bool, "Окно с настройками.MCC (UE Mobile Country Code)"=w83:dbl, "Окно с настройками.MNC (UE Mobile Network Code)"=w82:dbl, "Окно с настройками.MSIN (Mobile Subscription ID)"=w81:dbl, "Окно с настройками.Call Release Type"=w80:u16, "Окно с настройками.InputScaleFactor"=w79:u16, "Окно с настройками.OutputScaleFactor"=w78:u16, "Окно с настройками.Post MSD wave file playback 3GPP  26.269 \nEU_DTMF_tones"=w77:bool, "Окно с настройками.Scenario"=w76:u16, "Окно с настройками.AlAckBehavior"=w75:u16, "Окно с настройками.PSAP listens for PUSH"=w74:bool)
            n98 = property on="Номер образца" class="Ring (strict)"("Value"=w114) -> ()  [unwired: 2 in, 2 out]
            n99 = property on="Номер испытания" class="Ring (strict)"("Value"=w113) -> ()  [unwired: 2 in, 2 out]
            n100 = property on="Условия окружающей среды" class="Ring (strict)"("Value"=w112) -> ()  [unwired: 2 in, 2 out]
            n101 = property on="Источник питания" class="Ring (strict)"("Value"=w111) -> ()  [unwired: 2 in, 2 out]
            n102 = property on="Напряжение источника" class="Ring (strict)"("Value"=w110) -> ()  [unwired: 2 in, 2 out]
            n103 = property on="Режим звонка связь" class="Ring (strict)"("Value"=w109) -> ()  [unwired: 2 in, 2 out]
            n104 = property on="Аунтетификация" class="Ring (strict)"("Value"=w106) -> ()  [unwired: 2 in, 2 out]
            n105 = property on="Сим карта" class="Ring (strict)"("Value"=w104) -> ()  [unwired: 2 in, 2 out]
            n106 = property on="Количество повторов измерений" class="DigNum (strict)"("Value"=w105) -> ()  [unwired: 2 in, 2 out]
            n107 = property on="Режим звонка тональный модем" class="Ring (strict)"("Value"=w108) -> ()  [unwired: 2 in, 2 out]
            n108 = property on="Количество итераций TM" class="DigNum (strict)"("Value"=w107) -> ()  [unwired: 2 in, 2 out]
            n109 = property on="VISA adress of CMW500" class="Str"("Value"=w103) -> ()  [unwired: 2 in, 2 out]
            n110 = property on="Input attenuation" class="DigNum (strict)"("Value"=w102) -> ()  [unwired: 2 in, 2 out]
            n111 = property on="Output attenuation" class="DigNum (strict)"("Value"=w101) -> ()  [unwired: 2 in, 2 out]
            n112 = property on="GSM Band" class="Ring (strict)"("Value"=w100) -> ()  [unwired: 2 in, 2 out]
            n113 = property on="BCCH Channel Number" class="DigNum (strict)"("Value"=w73) -> ()  [unwired: 2 in, 2 out]
            n114 = property on="TCH Channel number" class="DigNum (strict)"("Value"=w99) -> ()  [unwired: 2 in, 2 out]
            n115 = property on="Codec" class="Ring (strict)"("Value"=w98) -> ()  [unwired: 2 in, 2 out]
            n116 = property on="AWGN" class="Ring (strict)"("Value"=w97) -> ()  [unwired: 2 in, 2 out]
            n117 = property on="snrRatioInDb" class="DigNum (strict)"("Value"=w96) -> ()  [unwired: 2 in, 2 out]
            n118 = property on="GSM Fading" class="Ring (strict)"("Value"=w95) -> ()  [unwired: 2 in, 2 out]
            n119 = property on="UL C/I ratio" class="Ring (strict)"("Value"=w94) -> ()  [unwired: 2 in, 2 out]
            n120 = property on="Use a custom network ID" class="Bool (strict)"("Value"=w93) -> ()  [unwired: 2 in, 2 out]
            n121 = property on="MCC (Mobile Country Code)" class="DigNum (strict)"("Value"=w92) -> ()  [unwired: 2 in, 2 out]
            n122 = property on="MNC (Mobile Network Code)" class="DigNum (strict)"("Value"=w91) -> ()  [unwired: 2 in, 2 out]
            n123 = property on="MNC digit count" class="Ring (strict)"("Value"=w90) -> ()  [unwired: 2 in, 2 out]
            n124 = property on="NCC (Network Color Code)" class="DigNum (strict)"("Value"=w89) -> ()  [unwired: 2 in, 2 out]
            n125 = property on="BCC (Base station Color Code)" class="DigNum (strict)"("Value"=w88) -> ()  [unwired: 2 in, 2 out]
            n126 = property on="LAC (Location Area Code)" class="DigNum (strict)"("Value"=w87) -> ()  [unwired: 2 in, 2 out]
            n127 = property on="RAC (Routing Area Code)" class="DigNum (strict)"("Value"=w86) -> ()  [unwired: 2 in, 2 out]
            n128 = property on="Cell Identity" class="DigNum (strict)"("Value"=w85) -> ()  [unwired: 2 in, 2 out]
            n129 = property on="Override UE ID" class="Bool (strict)"("Value"=w84) -> ()  [unwired: 2 in, 2 out]
            n130 = property on="MCC (UE Mobile Country Code)" class="DigNum (strict)"("Value"=w83) -> ()  [unwired: 2 in, 2 out]
            n131 = property on="MNC (UE Mobile Network Code)" class="DigNum (strict)"("Value"=w82) -> ()  [unwired: 2 in, 2 out]
            n132 = property on="MSIN (Mobile Subscription ID)" class="DigNum (strict)"("Value"=w81) -> ()  [unwired: 2 in, 2 out]
            n133 = property on="Call Release Type" class="Ring (strict)"("Value"=w80) -> ()  [unwired: 2 in, 2 out]
            n134 = property on="InputScaleFactor" class="Ring (strict)"("Value"=w79) -> ()  [unwired: 2 in, 2 out]
            n135 = property on="OutputScaleFactor" class="Ring (strict)"("Value"=w78) -> ()  [unwired: 2 in, 2 out]
            n136 = property on="Post MSD wave file playback 3GPP  26.269 EU_DTMF_tones" class="Bool (strict)"("Value"=w77) -> ()  [unwired: 2 in, 2 out]
            n137 = property on="Scenario" class="Ring (strict)"("Value"=w76) -> ()  [unwired: 2 in, 2 out]
            n138 = property on="AlAckBehavior" class="Ring (strict)"("Value"=w75) -> ()  [unwired: 2 in, 2 out]
            n139 = property on="PSAP listens for PUSH" class="Bool (strict)"("Value"=w74) -> ()  [unwired: 2 in, 2 out]
            n140 = property on="BCCH Channel Power" class="DigNum (strict)"("Value"=w72) -> ()  [unwired: 2 in, 2 out]
            n141 = property on="TCH Channel Power" class="DigNum (strict)"("Value"=w71) -> ()  [unwired: 2 in, 2 out]
          }
        }
      }
      frame "Apply values" {
        n142 = flat-sequence {
          tunnel: ["InputScaleFactor"] -> w124
          tunnel: ["OutputScaleFactor"] -> w123
          tunnel: ["Post MSD wave file playback 3GPP  26.269 EU_DTMF_tones"] -> w122
          tunnel: ["Scenario"] -> w121
          tunnel: ["AlAckBehavior"] -> w120
          tunnel: ["PSAP listens for PUSH"] -> w119
          frame #0 {
            # "PSAP"
          }
        }
        n143 = flat-sequence {
          tunnel: [w193] -> w145
          tunnel: [w192] -> w118
          tunnel: [w191] -> w144
          tunnel: [w190] -> w143
          tunnel: [w189] -> w142
          tunnel: [w188] -> w141
          tunnel: [w187] -> w140
          tunnel: [w186] -> w139
          tunnel: [w185] -> w138
          tunnel: [w184] -> w137
          tunnel: [w183] -> w136
          tunnel: [w182] -> w135
          tunnel: [w181] -> w134
          tunnel: [w180] -> w133
          tunnel: [w179] -> w132
          tunnel: [w178] -> w131
          tunnel: [w177] -> w130
          tunnel: [w176] -> w129
          tunnel: [w175] -> w128
          tunnel: [w174] -> w127
          tunnel: [w173] -> w126
          tunnel: [w172] -> w125
          tunnel: [w171] -> w117
          tunnel: [w170] -> w116
          frame #0 {
            # "GSM"
            n144 = flat-sequence {
              tunnel: ["GSM Band"] -> w193
              tunnel: ["BCCH Channel Number"] -> w192
              tunnel: ["TCH Channel number"] -> w191
              tunnel: ["Codec"] -> w190
              tunnel: ["AWGN"] -> w189
              tunnel: ["snrRatioInDb"] -> w188
              tunnel: ["GSM Fading"] -> w187
              tunnel: ["UL C/I ratio"] -> w186
              tunnel: ["BCCH Channel Power"] -> w171
              tunnel: ["TCH Channel Power"] -> w170
              frame #0 {
                # "GSM Band/AWGN"
              }
            }
            n145 = flat-sequence {
              tunnel: ["Use a custom network ID"] -> w185
              tunnel: ["MCC (Mobile Country Code)"] -> w184
              tunnel: ["MNC (Mobile Network Code)"] -> w183
              tunnel: ["MNC digit count"] -> w182
              tunnel: ["NCC (Network Color Code)"] -> w181
              tunnel: ["BCC (Base station Color Code)"] -> w180
              tunnel: ["LAC (Location Area Code)"] -> w179
              tunnel: ["RAC (Routing Area Code)"] -> w178
              tunnel: ["Cell Identity"] -> w177
              tunnel: ["Override UE ID"] -> w176
              tunnel: ["MCC (UE Mobile Country Code)"] -> w175
              tunnel: ["MNC (UE Mobile Network Code)"] -> w174
              tunnel: ["MSIN (Mobile Subscription ID)"] -> w173
              frame #0 {
                # "Custom network ID"
              }
            }
            n146 = flat-sequence {
              tunnel: ["Call Release Type"] -> w172
              frame #0 {
                # "Call Release Type"
              }
            }
          }
        }
        n147 = flat-sequence {
          tunnel: ["VISA adress of CMW500"] -> w151
          tunnel: ["Input attenuation"] -> w150
          tunnel: ["Output attenuation"] -> w149
          frame #0 {
            # "CMW500"
          }
        }
        n148 = flat-sequence {
          tunnel: ["Номер образца"] -> w159
          tunnel: ["Номер испытания"] -> w158
          tunnel: ["Условия окружающей среды"] -> w157
          tunnel: ["Источник питания"] -> w156
          tunnel: ["Напряжение источника"] -> w155
          tunnel: ["Режим звонка связь"] -> w154
          tunnel: ["Аунтетификация"] -> w153
          tunnel: ["Сим карта"] -> w152
          tunnel: ["Количество повторов измерений"] -> w148
          tunnel: ["Режим звонка тональный модем"] -> w147
          tunnel: ["Количество итераций TM"] -> w146
          frame #0 {
            # "Общие настройки"
          }
        }
        n149 = Bundle By Name(cluster=w161, "Окно с настройками.Номер образца"=w159, "Окно с настройками.Номер испытания"=w158, "Окно с настройками.Условия окружающей среды"=w157, "Окно с настройками.Источник питания"=w156, "Окно с настройками.Напряжение источника"=w155, "Окно с настройками.Режим звонка связь"=w154, "Окно с настройками.Аутентификация"=w153, "Окно с настройками.Сим карта"=w152, "Окно с настройками.Колличество повторов измерений"=w148, "Окно с настройками.Режим звонка тональный модем"=w147, "Окно с настройками.Количество итераций TM"=w146, "Окно с настройками.VISA adress of CMW500"=w151, "Окно с настройками.Input attenuation"=w150, "Окно с настройками.Output attenuation"=w149, "Окно с настройками.GSM Band"=w145, "Окно с настройками.BCCH Channel Power"=w117, "Окно с настройками.TCH Channel Power"=w116, "Окно с настройками.BCCH Channel Number"=w118, "Окно с настройками.TCH Channel Number"=w144, "Окно с настройками.Codec"=w143, "Окно с настройками.AWGN"=w142, "Окно с настройками.snrRatioInDb"=w141, "Окно с настройками.GSM Fading"=w140, "Окно с настройками.UL C/I ratio"=w139, "Окно с настройками.Use a custom network ID"=w138, "Окно с настройками.MCC (Mobile Country Code)"=w137, "Окно с настройками.MNC (Mobile Network Code)"=w136, "Окно с настройками.MNC digit count"=w135, "Окно с настройками.NCC (Network Color Code)"=w134, "Окно с настройками.BCC (Base station Color Code)"=w133, "Окно с настройками.LAC (Location Area Code)"=w132, "Окно с настройками.RAC (Routing Area Code)"=w131, "Окно с настройками.Cell Identity"=w130, "Окно с настройками.Override UE ID"=w129, "Окно с настройками.MCC (UE Mobile Country Code)"=w128, "Окно с настройками.MNC (UE Mobile Network Code)"=w127, "Окно с настройками.MSIN (Mobile Subscription ID)"=w126, "Окно с настройками.Call Release Type"=w125, "Окно с настройками.InputScaleFactor"=w124, "Окно с настройками.OutputScaleFactor"=w123, "Окно с настройками.Post MSD wave file playback 3GPP  26.269 \nEU_DTMF_tones"=w122, "Окно с настройками.Scenario"=w121, "Окно с настройками.AlAckBehavior"=w120, "Окно с настройками.PSAP listens for PUSH"=w119) -> (w160:T3)
      }
      frame "Stop" {
      }
    }
  }
  "CSMinfo out" <- w1
  "Error Out" <- w3
  n150 = while {
    tunnel: w5 -> [w235]
    stop <- w237 stop-if-true
    # "Event"
    n151 = event shown="[2] \"Применить\": Value Change" {
      selector: _ -> [_ _ _]
      dyn-events: _ -> [_ _ _]
      timeout: 1000 -> [_ _ _]
      tunnel: [_ TRUE TRUE] -> w237
      tunnel: w235 -> [_ w238 w243]
      event Timeout {
        n152 = event-data() -> ()  [unwired: 1 in, 3 out]
      }
      event Panel Close {
        n153 = event-data() -> ()  [unwired: 1 in, 4 out]
        n154 = call "MCUS_STM.vi"("StateMachineSteps"=T4[] [{"main stm"=enum."Stop", "data"=""}], "FNs"=enum16{"Back", "Front", "Replace"}."Replace", "Queue in"=w238) -> ()  [unwired: 7 in, 2 out]
      }
      event "Применить": Value Change {
        n155 = event-data() -> ()  [unwired: 1 in, 6 out]
        n156 = call "MCUS_STM.vi"("StateMachineSteps"=T4[] [{"main stm"=enum."Apply values", "data"=""}], "FNs"=enum16{"Back", "Front", "Replace"}."Back", "Queue in"=w243) -> ()  [unwired: 7 in, 2 out]
      }
    }
  }
